vi "get Last Error.vi"(8 "error in (no error)":errorcluster, 11 "pumpIndex":u32) -> (0 "error out":errorcluster, 3 "function return":string)   [LabVIEW 2018, in "AsiaPumpInterface.lvlib"]
doc: "extern ASIAPUMP_INTERFACE_API const char * getLastError(unsigned int pumpIndex );"
uses:
  <userlib>/AsiaPumpInterface/AsiaPumpInterface.lvlib
  <userlib>/AsiaPumpInterface/AsiaPumpInterface.dll
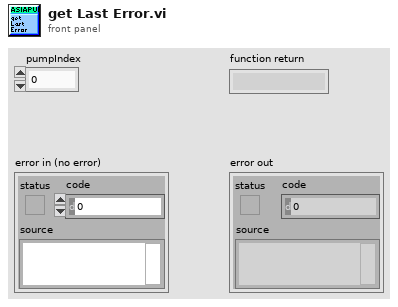
[diagram p1: front panel]
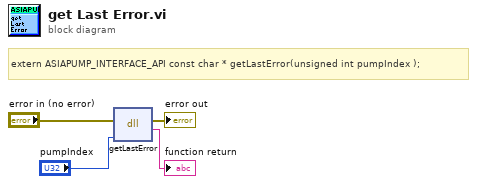
[diagram p0: block diagram]
diagram:
  # "extern ASIAPUMP_INTERFACE_API const char * getLastError(unsigned int pumpIndex );"
  n1 = dll-call lib="C:/Program Files (x86)/National Instruments/LabVIEW 2018/user.lib/AsiaPumpInterface/AsiaPumpInterface.*" fn="getLastError"(error in="error in (no error)", "pumpIndex"="pumpIndex") -> (error out=→"error out":errorcluster, →"function return":string)  [unwired: 3 in, 1 out]
